vi "Waitforfile.vi"() -> ()   [LabVIEW 2010]
panel:
  out "Complete?":bool
  in  "Incoming File":path
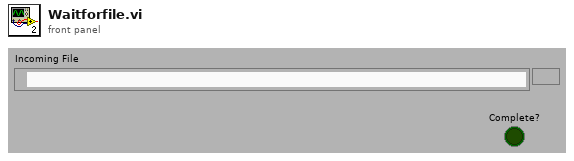
[diagram p1: front panel]
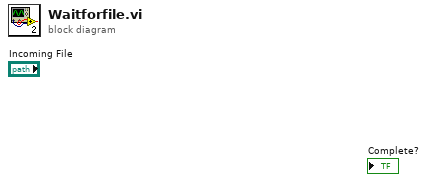
[diagram p0: block diagram]
diagram:
